vi "LTVDiffDriveCtrl_Pack_Tolerance.vi"(6 "Max Right Vel Tol M/S":dbl=0.15, 8 "Max Left Vel Tol M/S":dbl=0.15, 9 "Max Heading Tolerance Rad":dbl=0.6, 10 "Max Y Tolerance M":dbl=0.4, 11 "Max X Tolerance M":dbl=0.4) -> (3 "LTV_DiffDriveCtrl_Tolerance":T1={"Max Heading Tolerance Rad"=0.0, "Max X Tolerance M"=0.0, "Max Y Tolerance M"=0.0, "Max Left Vel Tol M/S"=0.2, "Max Right Vel Tol M/S"=0.2} {"Max Right Vel Tol M/S" format="%#_13g"; "Max Left Vel Tol M/S" format="%#_13g"; "Max Y Tolerance M" format="%#_13g"; "Max X Tolerance M" format="%#_13g"; "Max Heading Tolerance Rad" format="%#_13g"})   [LabVIEW 2019, in "Trajectory_Library.lvlib"]
uses:
  Trajectory_Library.lvlib
  TypeDef/LTV_DIFF_DRIVE_CTRL_TOLERANCE.CTL
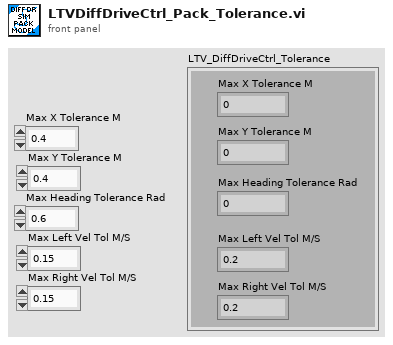
[diagram p1: front panel]
types:
  T1 = typedef "Trajectory_Library.lvlib/LTV_DIFF_DRIVE_CTRL_TOLERANCE.CTL" = cluster{"Max Heading Tolerance Rad":dbl, "Max X Tolerance M":dbl, "Max Y Tolerance M":dbl, "Max Left Vel Tol M/S":dbl, "Max Right Vel Tol M/S":dbl}
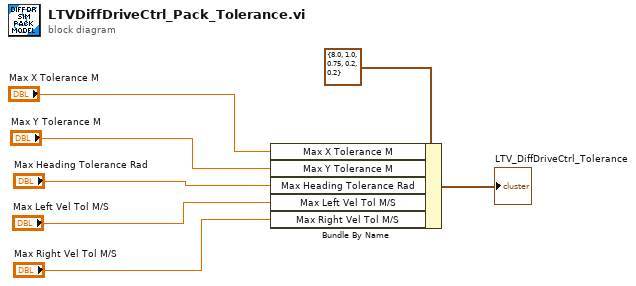
[diagram p0: block diagram]
diagram:
  n1 = Bundle By Name(cluster=T1 {"Max Heading Tolerance Rad"=8.0, "Max X Tolerance M"=1.0, "Max Y Tolerance M"=0.75, "Max Left Vel Tol M/S"=0.2, "Max Right Vel Tol M/S"=0.2} ("SngJntArmSim_Simulation _Params"), "Max X Tolerance M"="Max X Tolerance M", "Max Y Tolerance M"="Max Y Tolerance M", "Max Heading Tolerance Rad"="Max Heading Tolerance Rad", "Max Left Vel Tol M/S"="Max Left Vel Tol M/S", "Max Right Vel Tol M/S"="Max Right Vel Tol M/S") -> (→"LTV_DiffDriveCtrl_Tolerance":T1)
